vi "删除数组成员.vi"() -> ()   [LabVIEW 2010]
panel:
  out "被删除的部分":dbl[][](array[numeric]) format="%.2f"
  out "删除元素后的数组":dbl[][](array[numeric]) format="%.2f"
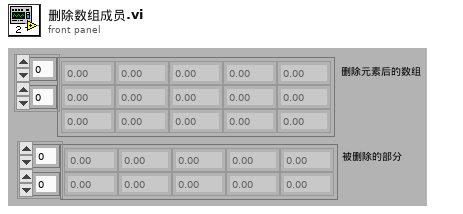
[diagram p1: front panel]
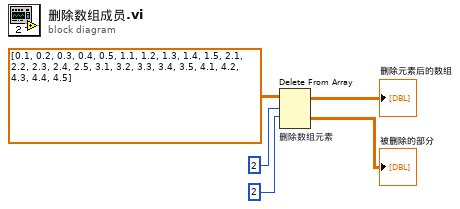
[diagram p0: block diagram]
diagram:
  n1 = Delete From Array "删除数组元素"(array=dbl[][] [[0.1, 0.2, 0.3, 0.4, 0.5], [1.1, 1.2, 1.3, 1.4, 1.5], [2.1, 2.2, 2.3, 2.4, 2.5], [3.1, 3.2, 3.3, 3.4, 3.5], [4.1, 4.2, 4.3, 4.4, 4.5]], length=2 ("disabled index (row)"), index (row)=2) -> (deleted portion=→"被删除的部分":dbl[][], array with subset deleted=→"删除元素后的数组":dbl[][])  [unwired: 1 in]
